vi "Erase Tx.vi"(8 "error in (no error)":errorcluster, 11 "RxTx in":refnum<class "CM_RxTx.lvclass">) -> (0 "error out":errorcluster, 3 "RxTx out":refnum<class "CM_RxTx.lvclass">)   [LabVIEW 2018, in "CM_RxTx.lvclass"]
doc: "Erase Tx message"
uses:
  CM_RxTx.lvclass
  CM_RxTx.lvclass/CM_RxTx.ctl
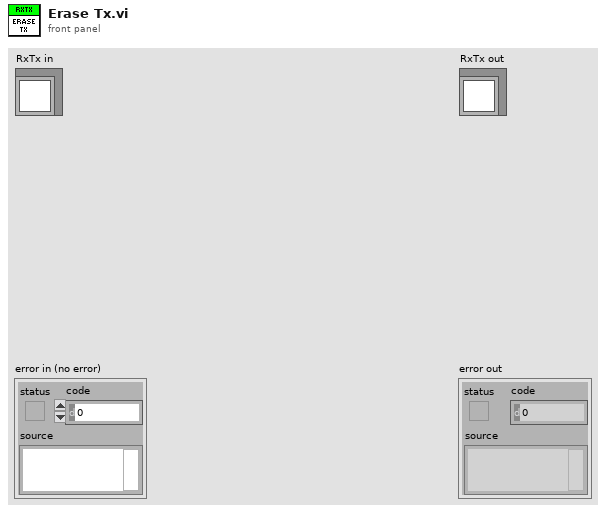
[diagram p1: front panel]
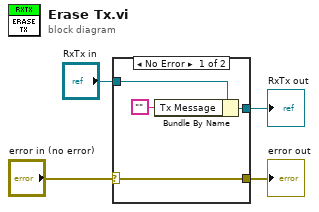
[diagram p0: block diagram]
diagram:
  n1 = case shown="No Error" "error in (no error)" {
    selector: "error in (no error)" -> [w8 w10]
    tunnel: [w8 w10] -> w3
    tunnel: [w6 w9] -> w1
    tunnel: "RxTx in" -> [w7 w9]
    frame No Error {
      n2 = Bundle By Name(cluster=w7, "Tx Message"="") -> (w6:refnum<class "CM_RxTx.lvclass">)
    }
    frame Error {
    }
  }
  "error out" <- w3
  "RxTx out" <- w1
